vi "subDAQ_SetFilterSet.vi"(6 "Ti-E cluster":T3, 7 "Filterset cluster":T1={"filter set (row)"=9, "Light control ref"=refnum, "Confocal Refnum"=refnum, "DAQ ports"={"Lasers DO lines"=["Dev2/port0/line0", "Dev2/port0/line1", "Dev2/port0/line2", "Dev2/port0/line3", "Dev2/port0/line4", "Dev2/port0/line5"], "Lasers AO lines"=["Dev2/ao0", "Dev2/ao1", "Dev2/ao2", "Dev2/ao3", "Dev2/ao4", "Dev2/ao5"], "Patch AO line"="Dev1/ao1", "Patch AI lines 1"={"Patch scaled output"="Dev1/ai13", "Patch 10 V_m "="Dev1/ai8"}, "Camera timing DI"="Dev1/port0/line8", "Dev1 timing DO "="Dev1/port0/line9", "Dev1 trigger source"="/Dev1/PFI0", "Dev2 trigger source"="/Dev2/PFI0", "LED line"="Dev1/port0/line0", "Global Shutter line"="Dev2/port0/line6", "Patch AI lines 2"={"Cell capacitance"="Dev1/ai9", "Mode"="Dev1/ai10", "Frequency"="Dev1/ai11", "Gain"="Dev1/ai12"}}, "Confocal VISA Setting"="COM1"}, 8 "error in":errorcluster) -> (0 "error out":errorcluster)   [LabVIEW 2015]
uses:
  <vilib>/Analysis/Matrix/Datatypes/RealMatrix.ctl
  <vilib>/Analysis/Matrix/NI_Matrix.lvlib
panel:
  out "Light control":T2={"Filter Set"=9, "Lasers DO"=[FALSE, TRUE, FALSE, FALSE, FALSE, FALSE], "Lasers AO (V)"=[1.94, 2.0, 2.0, 5.0, 4.0, 0.0], "LED"=FALSE, "Global"=FALSE} {"Lasers AO (V)" min=0.0 max=5.0 step=0.01 scale=0.0..5.0 scale format="%#1.2f"; "Filter Set" items=["R-QuasAr", "R-Cy5", "R-mCherry", "R-mOrange", "R-GFP", "R-CFP/DAPI", "R-BFP", "R-LED", "SDC-Cy5", "SDC-mCherry", "SDC-mO2", "SDC-GFP", "SDC-CFP/DAPI", "SDC-BFP", "SDC-LED"]}
  in  "Filter Set Table":T4=[[0.0, 5.0, 2.0, 1.0, 0.0, 1.0, 0.0], [1.0, 0.0, 2.0, 1.0, 0.0, 1.0, 0.0], [2.0, 1.0, 2.0, 2.0, 0.0, 1.0, 0.0], [3.0, 2.0, 1.0, 3.0, 0.0, 1.0, 0.0], [4.0, 3.0, 2.0, 6.0, 0.0, 1.0, 0.0], [5.0, 4.0, 2.0, 5.0, 0.0, 1.0, 0.0], [6.0, 4.0, 2.0, 5.0, 0.0, 1.0, 0.0], [7.0, -1.0, 6.0, 4.0, 0.0, 0.0, 1.0], [8.0, 0.0, 3.0, 4.0, 4.0, 0.0, 0.0], [9.0, 1.0, 3.0, 4.0, 3.0, 0.0, 0.0], [10.0, 2.0, 3.0, 4.0, 5.0, 0.0, 0.0], [11.0, 2.0, 3.0, 4.0, 2.0, 0.0, 0.0], [12.0, 4.0, 3.0, 4.0, 1.0, 0.0, 0.0], [13.0, 4.0, 3.0, 4.0, 1.0, 0.0, 0.0], [14.0, -1.0, 6.0, 4.0, 6.0, 0.0, 1.0], [15.0, 3.0, 3.0, 4.0, 3.0, 0.0, 0.0], [16.0, 3.0, 3.0, 4.0, 4.0, 0.0, 0.0]]
  # "Change Filter set according to the Table"
  # "Filter Set Table"
  # "No.    Laser   Top    Btm     FW     Glb    LED"
  # "Red"
  # "637"
  # "561"
  # "488"
  # "405"
  # "532"
  # "637"
  # "561"
  # "532"
  # "488"
  # "405"
  # "Red"
  # "Red"
  # "637"
  # "561"
  # "488"
  # "405"
  # "532"
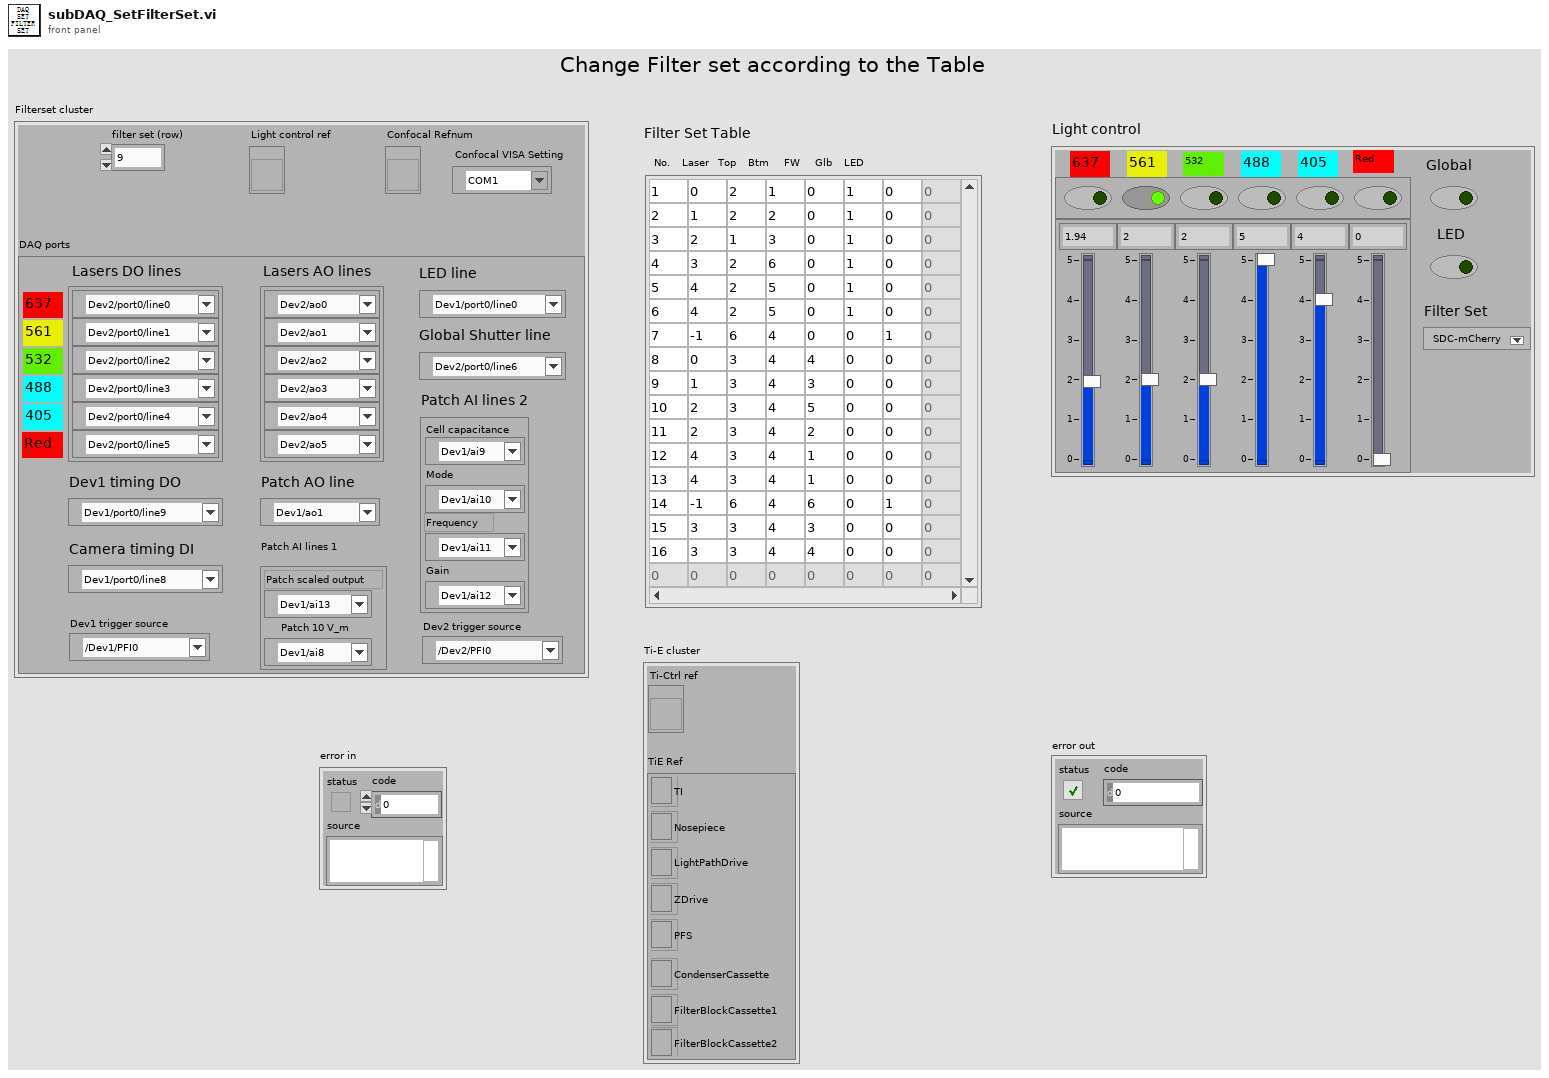
[diagram p1: front panel]
types:
  T1 = cluster{"filter set (row)":i32, "Light control ref":refnum<vi>, "Confocal Refnum":refnum<vi>, "DAQ ports":cluster{"Lasers DO lines":tag[], "Lasers AO lines":tag[], "Patch AO line":tag, "Patch AI lines 1":cluster{"Patch scaled output":tag, "Patch 10 V_m ":tag}, "Camera timing DI":tag, "Dev1 timing DO ":tag, "Dev1 trigger source":tag, "Dev2 trigger source":tag, "LED line":tag, "Global Shutter line":tag, "Patch AI lines 2":cluster{"Cell capacitance":tag, "Mode":tag, "Frequency":tag, "Gain":tag}}, "Confocal VISA Setting":refnum<visa-resource-name>}
  T2 = cluster{"Filter Set":i32, "Lasers DO":bool[], "Lasers AO (V)":dbl[], "LED":bool, "Global":bool}
  T3 = cluster{"Ti-Ctrl ref":refnum<vi>, "TiE Ref":cluster{"TI":refnum<k7>, "Nosepiece":refnum<k7>, "LightPathDrive":refnum<k7>, "ZDrive":refnum<k7>, "PFS":refnum<k7>, "CondenserCassette":refnum<k7>, "FilterBlockCassette1":refnum<k7>, "FilterBlockCassette2":refnum<k7>}}
  T4 = typedef "NI_Matrix.lvlib/RealMatrix.ctl" = dbl[][]
  T5 = cluster{"SDC shutter":bool, "Filter wheel":u16, "FW speed":i32, "Disk spinning":bool, "Disk speed (rpm)":dbl}
  T6 = cluster{"Obj":u16, "Cube Bottom":u16, "Cube Top":u16, "PFS-Ctrl":cluster{"PFS IO":bool, "PSF Err":bool, "PSF Pos":u32}, "Z-Ctrl":cluster{"Z-pos":dbl, "Home":bool, "Sensitivity":u8}, "Condenser":u16, "Lightpath":enum32{"EYE", "L100", "R100", "L80"}}
  T7 = cluster{"TI":refnum<k7>, "Nosepiece":refnum<k7>, "LightPathDrive":refnum<k7>, "ZDrive":refnum<k7>, "PFS":refnum<k7>, "CondenserCassette":refnum<k7>, "FilterBlockCassette1":refnum<k7>, "FilterBlockCassette2":refnum<k7>}
  T8 = cluster{"Lasers DO lines":tag[], "Lasers AO lines":tag[], "Patch AO line":tag, "Patch AI lines 1":cluster{"Patch scaled output":tag, "Patch 10 V_m ":tag}, "Camera timing DI":tag, "Dev1 timing DO ":tag, "Dev1 trigger source":tag, "Dev2 trigger source":tag, "LED line":tag, "Global Shutter line":tag, "Patch AI lines 2":cluster{"Cell capacitance":tag, "Mode":tag, "Frequency":tag, "Gain":tag}}
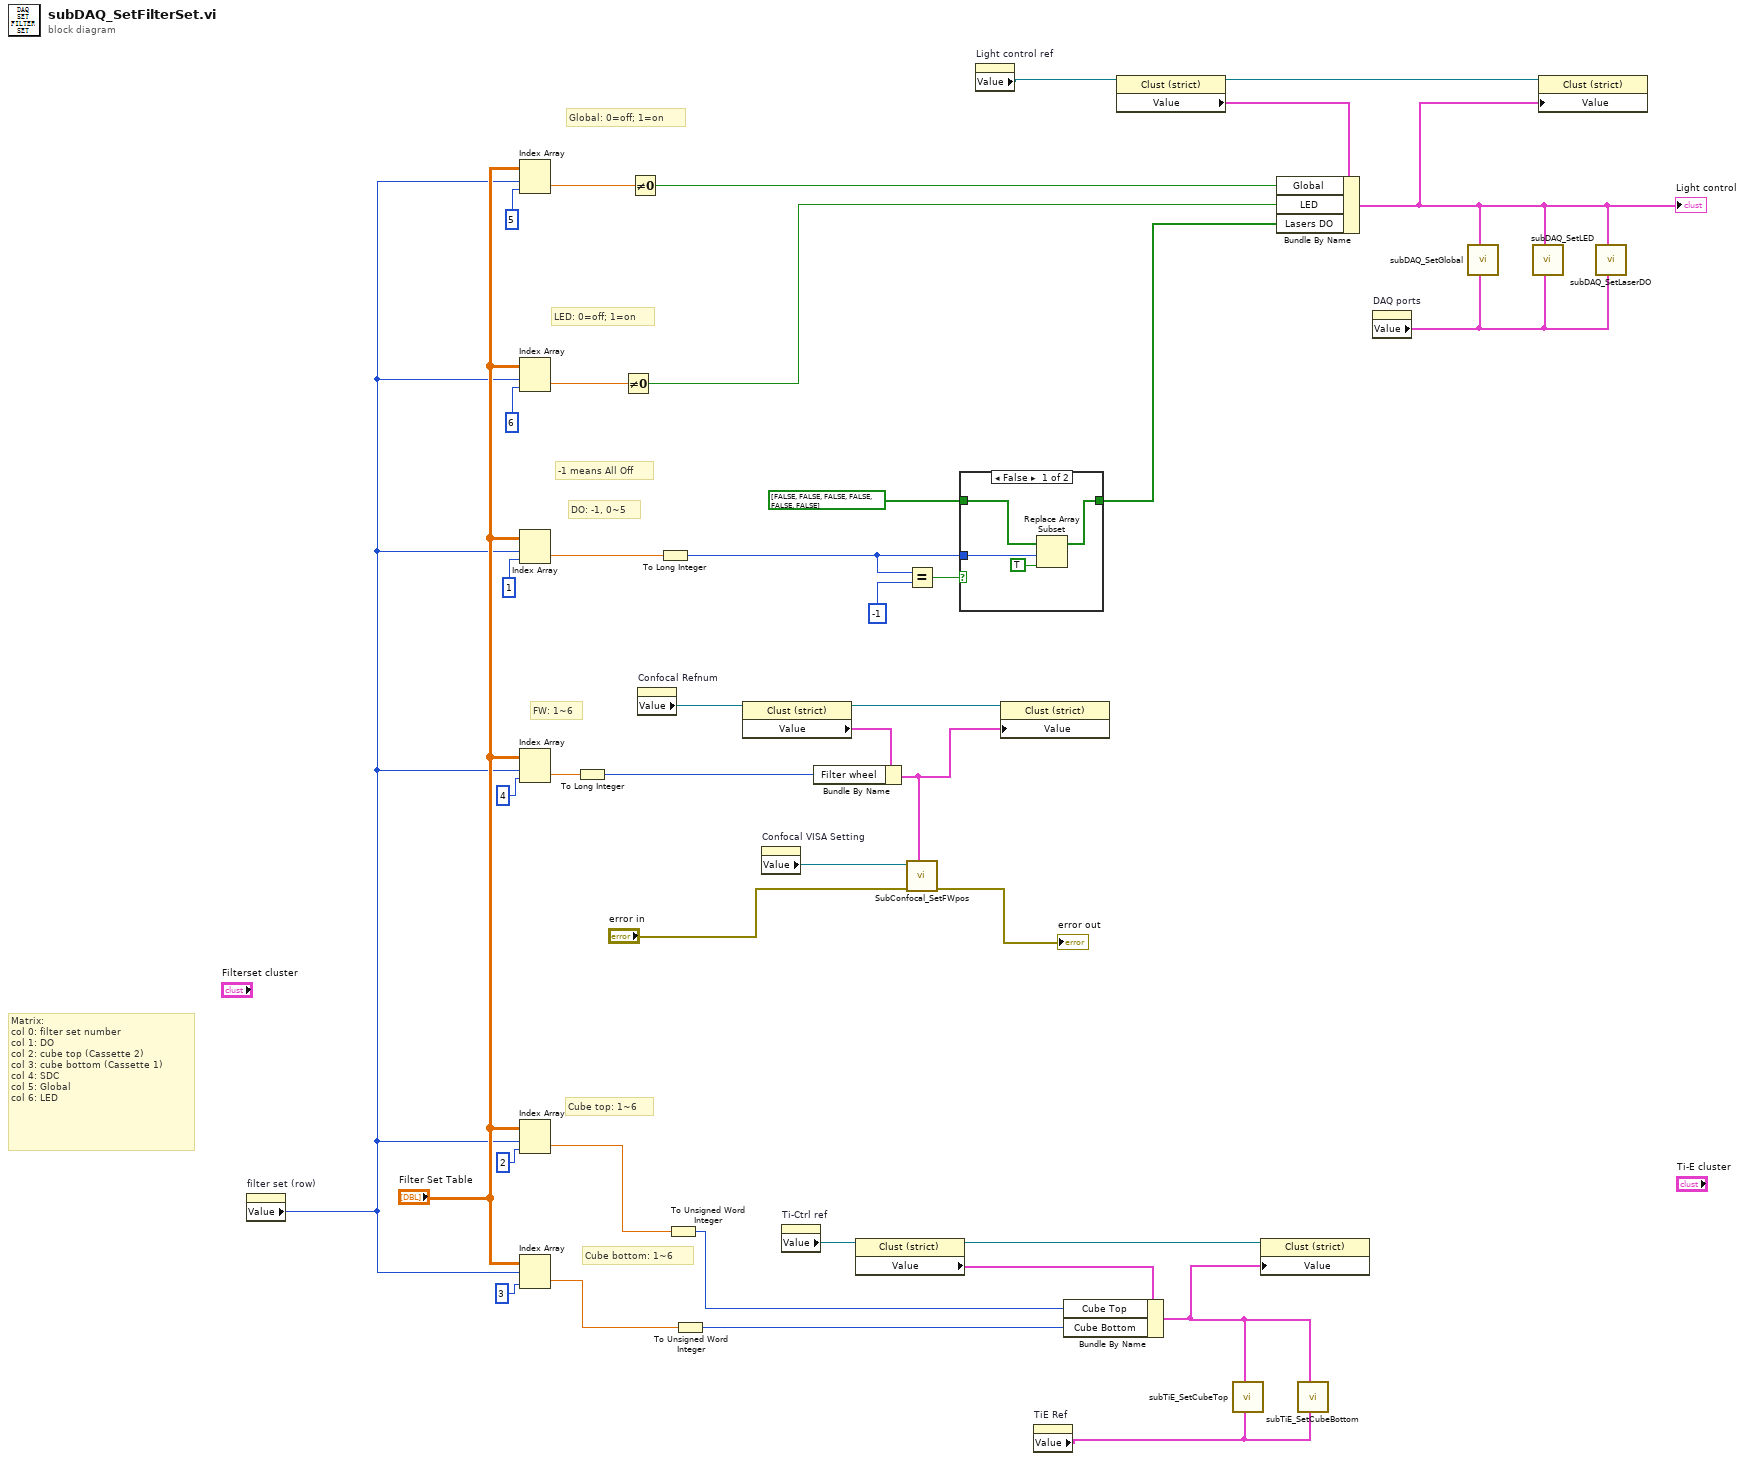
[diagram p0: block diagram]
diagram:
  # "-1 means All Off"
  # "LED: 0=off; 1=on"
  # "Global: 0=off; 1=on"
  # "FW: 1~6"
  # "Cube bottom: 1~6"
  # "Cube top: 1~6"
  # "DO: -1, 0~5"
  # "Matrix:\ncol 0: filter set number\ncol 1: DO\ncol 2: cube top (Cassette 2)\ncol 3: cube bottom (Cassette 1)\ncol 4: SDC\ncol 5: Global\ncol 6: LED"
  n1 = property on="filter set (row)" class="DigNum (strict)"() -> ("Value"=w7:i32)  [unwired: 2 in, 2 out]
  n2 = Index Array(array="Filter Set Table", index (row)=w7, index (col)=5) -> (element=w27:dbl)
  n3 = Index Array(array="Filter Set Table", index (row)=w7, index (col)=6) -> (element=w24:dbl)
  n4 = Index Array(array="Filter Set Table", index (row)=w7, index (col)=1) -> (element=w38:dbl)
  n5 = Index Array(array="Filter Set Table", index (row)=w7, index (col)=4) -> (element=w31:dbl)
  n6 = Index Array(array="Filter Set Table", index (row)=w7, index (col)=2) -> (element=w34:dbl)
  n7 = Index Array(array="Filter Set Table", index (row)=w7, index (col)=3) -> (element=w33:dbl)
  n8 = To Long Integer(number=w31) -> (32bit integer=w15:i32)
  n9 = Not Equal To 0?(x=w24) -> (x != 0?=w20:bool)
  n10 = Not Equal To 0?(x=w27) -> (x != 0?=w21:bool)
  n11 = property on="Confocal Refnum" class="LVObjRef (strict)"() -> ("Value"=w9:refnum<vi>)  [unwired: 2 in, 2 out]
  n12 = To Long Integer(number=w38) -> (32bit integer=w28:i32)
  n13 = To Unsigned Word Integer(number=w34) -> (unsigned 16bit integer=w4:u16)
  n14 = To Unsigned Word Integer(number=w33) -> (unsigned 16bit integer=w3:u16)
  n15 = property class="Clust (strict)"(reference=w9) -> (reference out=w14:refnum<vi>, "Value"=w16:T5)  [unwired: 1 in, 1 out]
  n16 = property on="Confocal VISA Setting" class="VISAName"() -> ("Value"=w8:refnum<visa-resource-name>)  [unwired: 2 in, 2 out]
  n17 = property on="Ti-Ctrl ref" class="LVObjRef (strict)"() -> ("Value"=w12:refnum<vi>)  [unwired: 2 in, 2 out]
  n18 = Bundle By Name(cluster=w16, "Filter wheel"=w15) -> (w13:T5)
  n19 = property class="Clust (strict)"(reference=w12) -> (reference out=w6:refnum<vi>, "Value"=w5:T6)  [unwired: 1 in, 1 out]
  n20 = Equal?(x=w28, y=-1) -> (x = y?=w30:bool)
  n21 = call "SubConfocal_SetFWpos.vi"("Confocal scanner"=w13, "Error In"="error in", "Confocal line (VISA IN)"=w8) -> ("Error out"=→"error out":errorcluster)  [unwired: 7 in, 1 out]
  n22 = case shown="False" w30 {
    tunnel: bool[] [FALSE, FALSE, FALSE, FALSE, FALSE, FALSE] ("initialized array") -> [w45 w46]
    tunnel: [w43 w46] -> w17
    tunnel: w28 -> [w42 _]
    frame False {
      n23 = Replace Array Subset(array=w45, new element=TRUE ("new element/subarray"), index=w42) -> (w43:bool[])
    }
    frame True {
      # "All OFF"
    }
  }
  n24 = property on="Light control ref" class="LVObjRef (strict)"() -> ("Value"=w11:refnum<vi>)  [unwired: 2 in, 2 out]
  n25 = property class="Clust (strict)"(reference=w14, "Value"=w13) -> ()  [unwired: 1 in, 2 out]
  n26 = property on="TiE Ref" class="Clust (strict)"() -> ("Value"=w2:T7)  [unwired: 2 in, 2 out]
  n27 = Bundle By Name(cluster=w5, "Cube Top"=w4, "Cube Bottom"=w3) -> (w1:T6)
  n28 = property class="Clust (strict)"(reference=w11) -> (reference out=w23:refnum<vi>, "Value"=w22:T2)  [unwired: 1 in, 1 out]
  n29 = call "subTiE_SetCubeTop.vi"("Ref"=w2, "TI-Ctrl"=w1) -> ()  [unwired: 10 in]
  n30 = property class="Clust (strict)"(reference=w6, "Value"=w1) -> ()  [unwired: 1 in, 2 out]
  n31 = Bundle By Name(cluster=w22, "Global"=w21, "LED"=w20, "Lasers DO"=w17) -> (w19:T2)
  "Light control" <- w19
  n32 = call "subTiE_SetCubeBottom.vi"("Ref"=w2, "TI-Ctrl"=w1) -> ()  [unwired: 10 in]
  n33 = property on="DAQ ports" class="Clust (strict)"() -> ("Value"=w10:T8)  [unwired: 2 in, 2 out]
  n34 = call "subDAQ_SetGlobal.vi"("DAQ ports"=w10, "Light control (All off)"=w19) -> ()  [unwired: 9 in, 1 out]
  n35 = call "subDAQ_SetLED.vi"("DAQ ports"=w10, "Light control (All Off)"=w19) -> ()  [unwired: 9 in, 1 out]
  n36 = property class="Clust (strict)"(reference=w23, "Value"=w19) -> ()  [unwired: 1 in, 2 out]
  n37 = call "subDAQ_SetLaserDO.vi"("DAQ ports"=w10, "Light control (All off)"=w19) -> ()  [unwired: 9 in, 1 out]
